vi "drawCurve.vi"(0 "reference":refnum<class "Graphics.lvclass">, 1 "StartPoint":T1 {"y" format="%.2f"; "x" format="%.2f"}, 2 "ControlPointStart":T1 {"y" format="%.2f"; "x" format="%.2f"}, 3 "ControlPointEnd":T1 {"y" format="%.2f"; "x" format="%.2f"}, 4 "EndPoint":T1 {"y" format="%.2f"; "x" format="%.2f"}, 5 "error in (no error)":errorcluster, 9 "color(if not used=default color)":u32=536870912 format="%.0x") -> (14 "reference out":refnum<class "Graphics.lvclass">, 19 "error out":errorcluster)   [LabVIEW 2020, in "Graphics.lvclass"]
uses:
  <resource>/Framework/Providers/Open_GDS/UML/Graphics_class/Graphics.lvclass
  <resource>/Framework/Providers/Open_GDS/UML/General/Point/Point Point2D.ctl
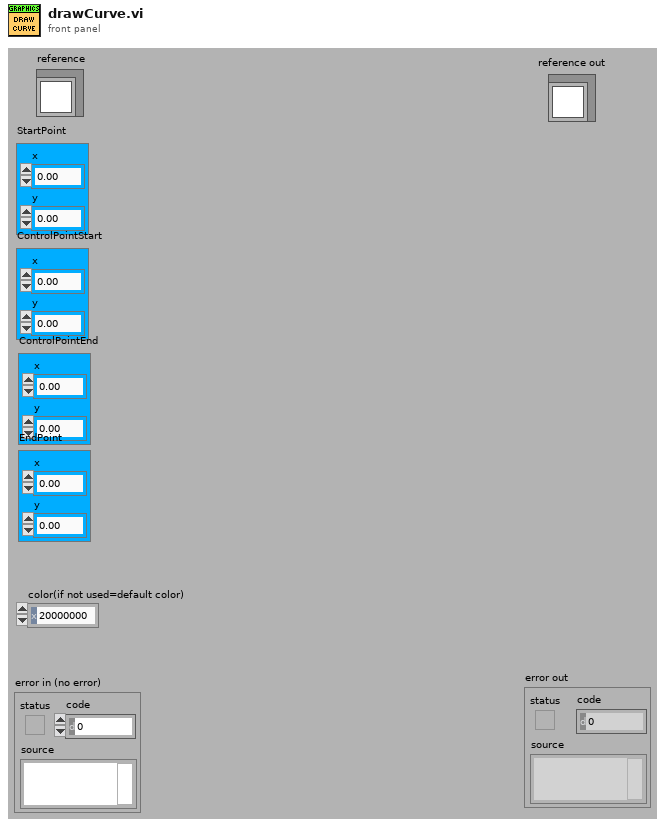
[diagram p1: front panel]
types:
  T1 = typedef "Point Point2D.ctl" = cluster{"x":dbl, "y":dbl}
  T2 = typedef "Graphics.lvclass/ObjectAttributes.ctl" = cluster{"drawColor":u32, "backgroundColor":u32, "font":T3, "fontType":T4, "picture":picture, "stroke":T5, "scaleX":dbl, "scaleY":dbl, "screenRef":refnum<vi>, "offsetX":dbl, "offsetY":dbl}
  T3 = typedef "Graphics.lvclass/FontType.ctl" = cluster{"Font Name:":string, "Size":i16, "Strikeout?":bool, "Italic?":bool, "Underline?":bool, "Outline?":bool, "Shadow?":bool, "Bold?":bool}
  T4 = typedef "Graphics.lvclass/LvFontType.ctl" = enum16{"User-specified Font", "Application Font", "System Font", "Dialog Font"}
  T5 = typedef "Graphics.lvclass/StrokeType.ctl" = enum16{"USE_DEFAULT", "SOLID", "DOTTED"}
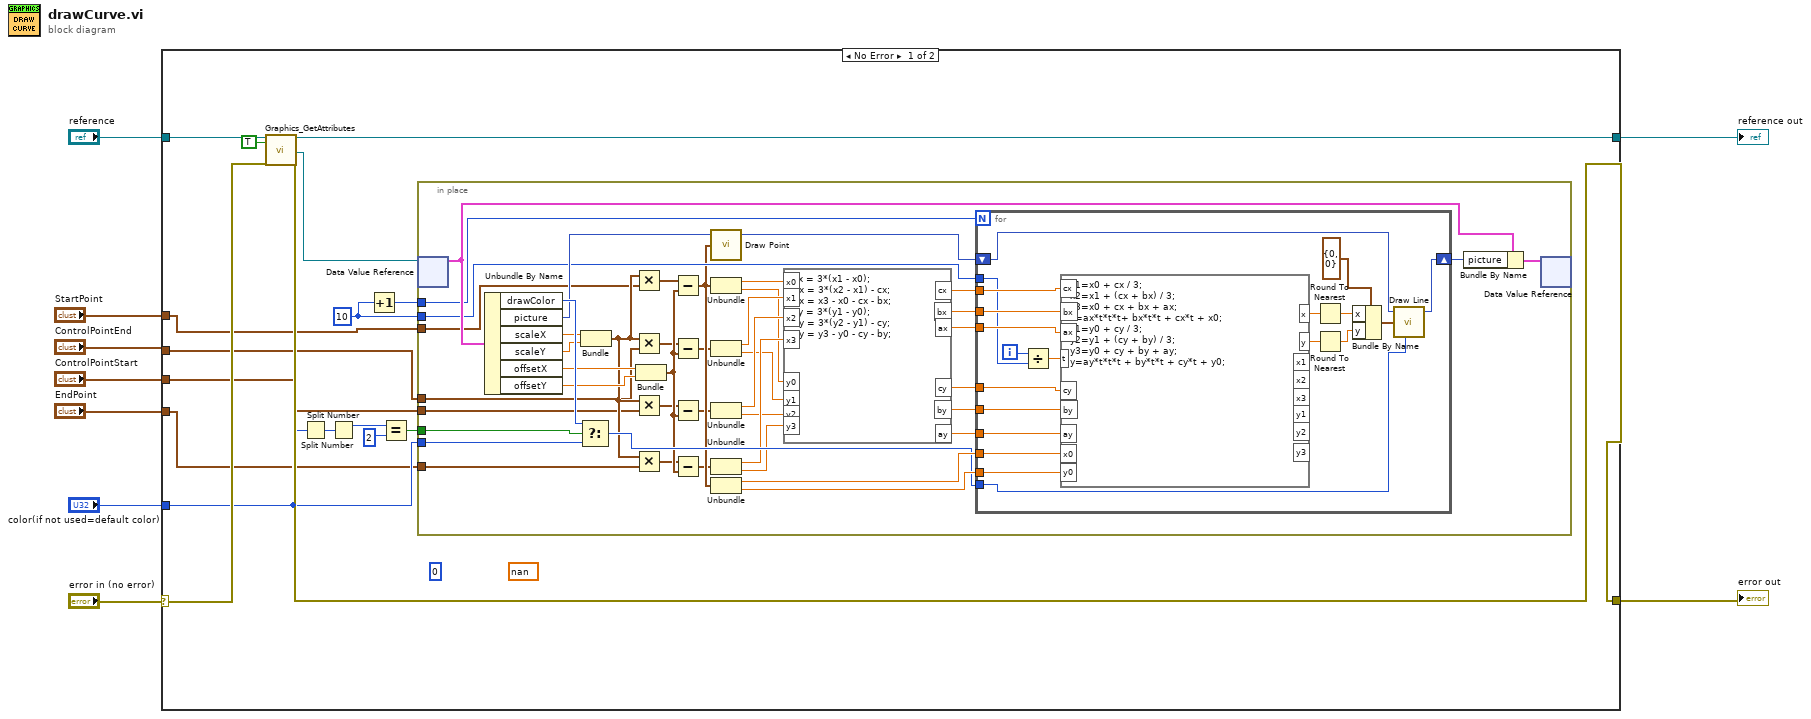
[diagram p0: block diagram]
diagram:
  n1 = case shown="No Error" "error in (no error)" {
    selector: "error in (no error)" -> [w20 w92]
    tunnel: "reference" -> [w26 w93]
    tunnel: [w25 w92] -> w8
    tunnel: [w24 w93] -> w7
    tunnel: "color(if not used=default color)" -> [w15 _]
    tunnel: "StartPoint" -> [w13 _]
    tunnel: "ControlPointEnd" -> [w12 _]
    tunnel: "ControlPointStart" -> [w11 _]
    tunnel: "EndPoint" -> [w10 _]
    frame No Error {
      (unwired) nan
      w16 = 10
      (unwired) 0
      n2 = call <resource>:"Graphics_GetAttributes.vi"("reference in"=w26, "OnlyGetDvrReference(False)"=TRUE, "error in (no error)"=w20) -> ("reference out"=w24:refnum<class "Graphics.lvclass">, "DataRef"=w18:refnum<data-value>, "error out"=w25:errorcluster)  [unwired: 13 in, 1 out]
      n3 = Split Number(x=w15) -> (hi(x)=w23:u16)  [unwired: 1 out]
      n4 = Split Number(x=w23) -> (hi(x)=w22:u8)  [unwired: 1 out]
      n5 = Increment(x=w16) -> (x+1=w17:i32)
      n6 = Equal?(x=w22, y=u8 2) -> (x = y?=w14:bool)
      n7 = in-place {
        in-place-border: w17 -> [w62]
        in-place-border: w16 -> [w58]
        in-place-border: w15 -> [w50]
        in-place-border: w14 -> [w49]
        in-place-border: w13 -> [w36]
        in-place-border: w12 -> [w35]
        in-place-border: w11 -> [w33]
        in-place-border: w10 -> [w31]
        n8 = in-place-dvr #1(w18) -> (w71:T2)  [unwired: 1 out]
        n9 = Unbundle By Name(w71) -> ("drawColor"=w68:u32, "picture"=w67:picture, "scaleX"=w66:dbl, "scaleY"=w65:dbl, "offsetX"=w64:dbl, "offsetY"=w63:dbl)
        n10 = Select(t=w68, s=w49, f=w50) -> (s? t:f=w51:u32)
        n11 = Bundle("scaleX"=w66, "scaleY"=w65) -> (w47:cluster{"scaleX":dbl, "scaleY":dbl})  [unwired: 1 out]
        n12 = Multiply(x=w47, y=w36) -> (x*y=w37:T1)
        n13 = Multiply(x=w47, y=w35) -> (x*y=w34:T1)
        n14 = Multiply(x=w47, y=w33) -> (x*y=w32:T1)
        n15 = Multiply(x=w47, y=w31) -> (x*y=w30:T1)
        n16 = Bundle("offsetX"=w64, "offsetY"=w63) -> (w46:cluster{"offsetX":dbl, "offsetY":dbl})  [unwired: 1 out]
        n17 = Subtract(x=w37, y=w46) -> (x-y=w48:T1)
        n18 = Subtract(x=w34, y=w46) -> (x-y=w27:T1)
        n19 = Subtract(x=w32, y=w46) -> (x-y=w28:T1)
        n20 = Subtract(x=w30, y=w46) -> (x-y=w29:T1)
        n21 = call <vilib>:"Draw Point.vi"("picture"=w67, "point(x,y)"=w48) -> ("new picture"=w57:picture)  [unwired: 2 in, 5 out]
        n22 = Unbundle(w48) -> ("x"=w45:dbl, "y"=w41:dbl)
        n23 = Unbundle(w27) -> ("x"=w44:dbl, "y"=w40:dbl)
        n24 = Unbundle(w28) -> ("x"=w43:dbl, "y"=w39:dbl)
        n25 = Unbundle(w29) -> ("x"=w42:dbl, "y"=w38:dbl)
        n26 = Unbundle(w48) -> ("x"=w53:dbl, "y"=w52:dbl)
        n27 = formula code="cx = 3*(x1 - x0);\nbx = 3*(x2 - x1) - cx;\nax = x3 - x0 - cx - bx;\ncy = 3*(y1 - y0);\nby = 3*(y2 - y1) - cy;\nay = y3 - y0 - cy - by;"("x0"=w45, "x1"=w44, "x2"=w43, "x3"=w42, "y0"=w41, "y1"=w40, "y2"=w39, "y3"=w38) -> ("cx"=w61:dbl, "bx"=w60:dbl, "ax"=w59:dbl, "cy"=w56:dbl, "by"=w55:dbl, "ay"=w54:dbl)
        n28 = for {
          N: w62 -> [_]
          tunnel: w61 -> [w91]
          tunnel: w60 -> [w90]
          tunnel: w59 -> [w89]
          tunnel: w58 -> [w87]
          shift-right: [w78] -> w70
          shift-left: w57 -> [w85]
          tunnel: w56 -> [w77]
          tunnel: w55 -> [w76]
          tunnel: w54 -> [w75]
          tunnel: w53 -> [w74]
          tunnel: w52 -> [w73]
          tunnel: w51 -> [w72]
          i -> [w88]
          n29 = Divide(x=w88, y=w87) -> (x/y=w86:dbl)
          n30 = formula code="x1=x0 + cx / 3;\nx2=x1 + (cx + bx) / 3;\nx3=x0 + cx + bx + ax;\nx=ax*t*t*t+ bx*t*t + cx*t + x0;\ny1=y0 + cy / 3;\ny2=y1 + (cy + by) / 3;\ny3=y0 + cy + by + ay;\ny=ay*t*t*t + by*t*t + cy*t + y0;"("cx"=w91, "bx"=w90, "ax"=w89, "t"=w86, "cy"=w77, "by"=w76, "ay"=w75, "x0"=w74, "y0"=w73) -> ("x"=w82:dbl, "y"=w81:dbl)  [unwired: 6 out]
          n31 = Round To Nearest(number=w82) -> (nearest integer value=w80:dbl)
          n32 = Round To Nearest(number=w81) -> (nearest integer value=w79:dbl)
          n33 = Bundle By Name(cluster=cluster{"x":i16, "y":i16} {"x"=0, "y"=0} ("end point"), "x"=w80, "y"=w79) -> (w83:cluster{"x":i16, "y":i16})
          n34 = call <vilib>:"Draw Line.vi"("picture"=w85, "end point"=w83, "color(black)"=w72) -> ("new picture"=w78:picture)  [unwired: 2 in, 4 out]
        }
        n35 = Bundle By Name(cluster=w71, "picture"=w70) -> (w69:T2)
        n36 = in-place-dvr #1(w69) -> ()  [unwired: 2 out]
      }
    }
    frame Error {
    }
  }
  "reference out" <- w7
  "error out" <- w8
